vi "Vision_0.vi"(8 "error in":errorcluster, 11 "Image In":T1) -> (0 "error out":errorcluster, 3 "Image Out":T1)   [LabVIEW 2016]
uses:
  <vilib>/vision/NI_Vision_Development_Module.lvlib
  <vilib>/vision/Image Controls.llb/IMAQ Image.ctl
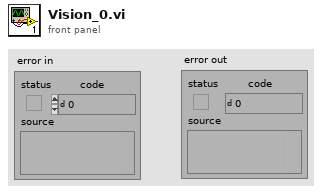
[diagram p1: front panel]
types:
  T1 = typedef "IMAQ Image.ctl" = refnum<image>
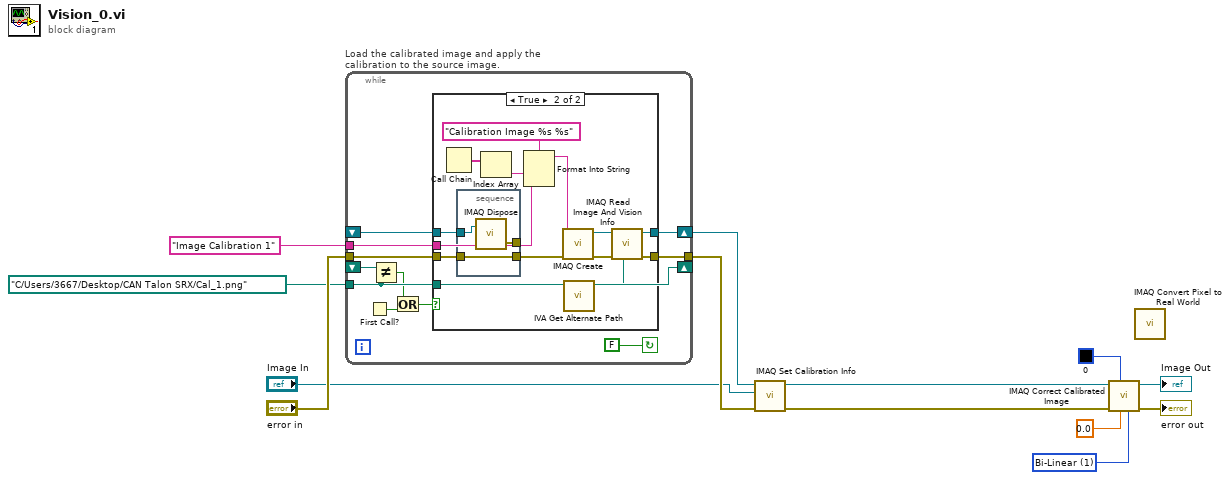
[diagram p0: block diagram]
diagram:
  w6 = u32 1 items=["Zero Order", "Bi-Linear", "Quadratic", "Cubic Spline"] ("Interpolation Type")
  n1 = while "Load the calibrated image and apply the calibration to the source image." {
    shift-right: [w24] -> w11
    shift-left: _ -> [w23]
    tunnel: [w21] -> w10
    tunnel: "error in" -> [w20]
    tunnel: path "C:/Users/3667/Desktop/CAN Talon SRX/Cal_1.png" ("File Path") -> [w17]
    tunnel: "Image Calibration 1" ("Step Name") -> [w19]
    shift-right: [w17] -> _
    shift-left: _ -> [w18]
    stop <- FALSE continue-if-true
    n2 = First Call?() -> (First Call?: T/F=w16:bool)
    n3 = Not Equal?(x=w18, y=w17) -> (x != y?=w15:bool)
    n4 = Or(x=w15, y=w16) -> (x .or. y?=w14:bool)
    n5 = case shown="True" w14 {
      tunnel: [w26 w38] -> w24
      tunnel: w23 -> [w26 w30]
      tunnel: [w25 w35] -> w21
      tunnel: w20 -> [w25 w31]
      tunnel: w17 -> [_ w28]
      tunnel: w19 -> [_ w32]
      frame False {
      }
      frame True {
        n6 = Call Chain() -> (call chain=w34:string[])
        n7 = stacked-sequence {
          tunnel: w31 -> [w42]
          tunnel: w30 -> [w43]
          tunnel: [w42] -> w29
          tunnel: [w41] -> _
          frame #0 {
            n8 = call "IMAQ Dispose"("Image"=w43) -> ("error out"=w41:errorcluster)  [unwired: 2 in, 3 out]
          }
        }
        n9 = Index Array(array=w34) -> (element=w33:string)  [unwired: 1 in]
        n10 = Format Into String(format string="Calibration Image %s %s" ("Image Name"), w33, w32) -> (resulting string=w40:string)  [unwired: 2 in, 1 out]
        n11 = call "IMAQ Create"("Image Name"=w40, "error in (no error)"=w29) -> ("New Image"=w37:T1, "error out"=w36:errorcluster)  [unwired: 2 in, 1 out]
        n12 = call <vilib>:"IVA Get Alternate Path.vi"("Path In"=w28) -> ("Path Out"=w27:path)  [unwired: 10 out]
        n13 = call "IMAQ Read Image And Vision Info"("File Path"=w27, "error in (no error)"=w36, "Image"=w37) -> ("error out"=w35:errorcluster, "Image Out"=w38:T1)  [unwired: 1 in, 6 out]
      }
    }
  }
  n14 = call "IMAQ Set Calibration Info"("error in (no error)"=w10, "Image Dst"="Image In", "Image Src"=w11) -> ("error out"=w9:errorcluster, "Calibrated Image"=w3:T1)  [unwired: 1 in, 6 out]
  n15 = call "IMAQ Correct Calibrated Image"("Interpolation Type"=w6, "Replace Value"=sgl 0.0, "Color Replace Value"=u32 0, "error in (no error)"=w9, "Image Src"=w3) -> ("error out"=→"error out":errorcluster, "Corrected Image"=→"Image Out":T1)  [unwired: 2 in, 3 out]
  n16 = call "IMAQ Convert Pixel to Real World"() -> ()  [unwired: 6 in, 6 out]
